vi "test_Read Cluster Register Value.vi"(8 "error in (no error)":errorcluster, 11 "TestCase in":refnum<class "FPGA Register IO Tests.lvclass">) -> (0 "error out":errorcluster, 3 "TestCase out":refnum<class "FPGA Register IO Tests.lvclass">)   [LabVIEW 2021, in "FPGA Register IO Tests.lvclass"]
uses:
  FPGA Register IO Tests.lvclass
  FPGA Register IO Tests.lvclass/FPGA Register IO Tests.ctl
  c83476ed-2beb-434a-be7f-ac9223862d10.vi
  APIs/FPGA Register IO/SubVIs/Parse Cluster Configuration.vi
  APIs/FPGA Register IO/Read Methods/Read Data Register/Instances/Read U8 Array.vi
  APIs/FPGA Register IO/SubVIs/Check Cluster Configuration Store.vi
  APIs/FPGA Register IO/Utilities/Find Register Offset.vi
  APIs/FPGA Register IO/SubVIs/Check Register Data Store.vi
  <userlib>/_OpenG.lib/lvdata/lvdata.llb/Variant to Header Info__ogtk.vi
  <userlib>/_OpenG.lib/lvdata/lvdata.llb/Split Cluster TD__ogtk.vi
  <userlib>/_OpenG.lib/lvdata/lvdata.llb/Cluster to Array of VData__ogtk.vi
  <vilib>/Utility/Data Type/Get Type Information.vi
  <userlib>/_OpenG.lib/lvdata/lvdata.llb/Get Strings from Enum__ogtk.vi
  APIs/FPGA Register IO/Error Handling/Error 6004.vi
  <vilib>/Utility/Data Type/Get Fixed-Point Information.vi
  APIs/FPGA Register IO/Error Handling/Error 6001.vi
  APIs/FPGA Register IO/Error Handling/Error 6000.vi
  APIs/FPGA Register IO/Error Handling/Error 6002.vi
  APIs/FPGA Register IO/Error Handling/Error 6003.vi
  <vilib>/FPGAPlugInAG/Dynamic/niLvFpga_Close_Dynamic.vi
  <vilib>/rvi/interface/nirviCloseFPGA/nirviCloseFPGA.xnode
  <vilib>/addons/_JKI Toolkits/VI Tester/TestCase.llb/TestCase.lvclass
  APIs/FPGA Register IO/FPGA Register IO.lvlib
  C:/Program Files/National Instruments/LabVIEW 2021/vi.lib/addons/_JKI Toolkits/VI Tester/TestCase.llb/TestCase.lvclass
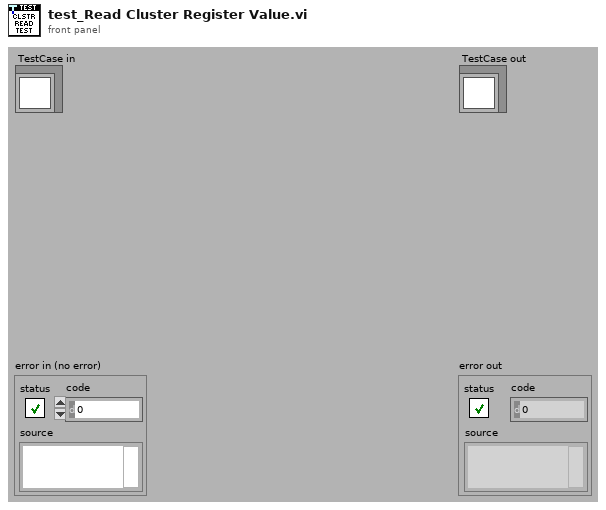
[diagram p1: front panel]
types:
  T1 = cluster{"I16":i16, "U64":u64, "SGL":sgl, "Bool":bool, "FXP 12/6":fxp<+/-,12,6>}
  T2 = cluster{"I16":i16, "U64":u64, "SGL":sgl, "Bool":bool, "FXP 12/6":fxp<+/-,12,6>}[]
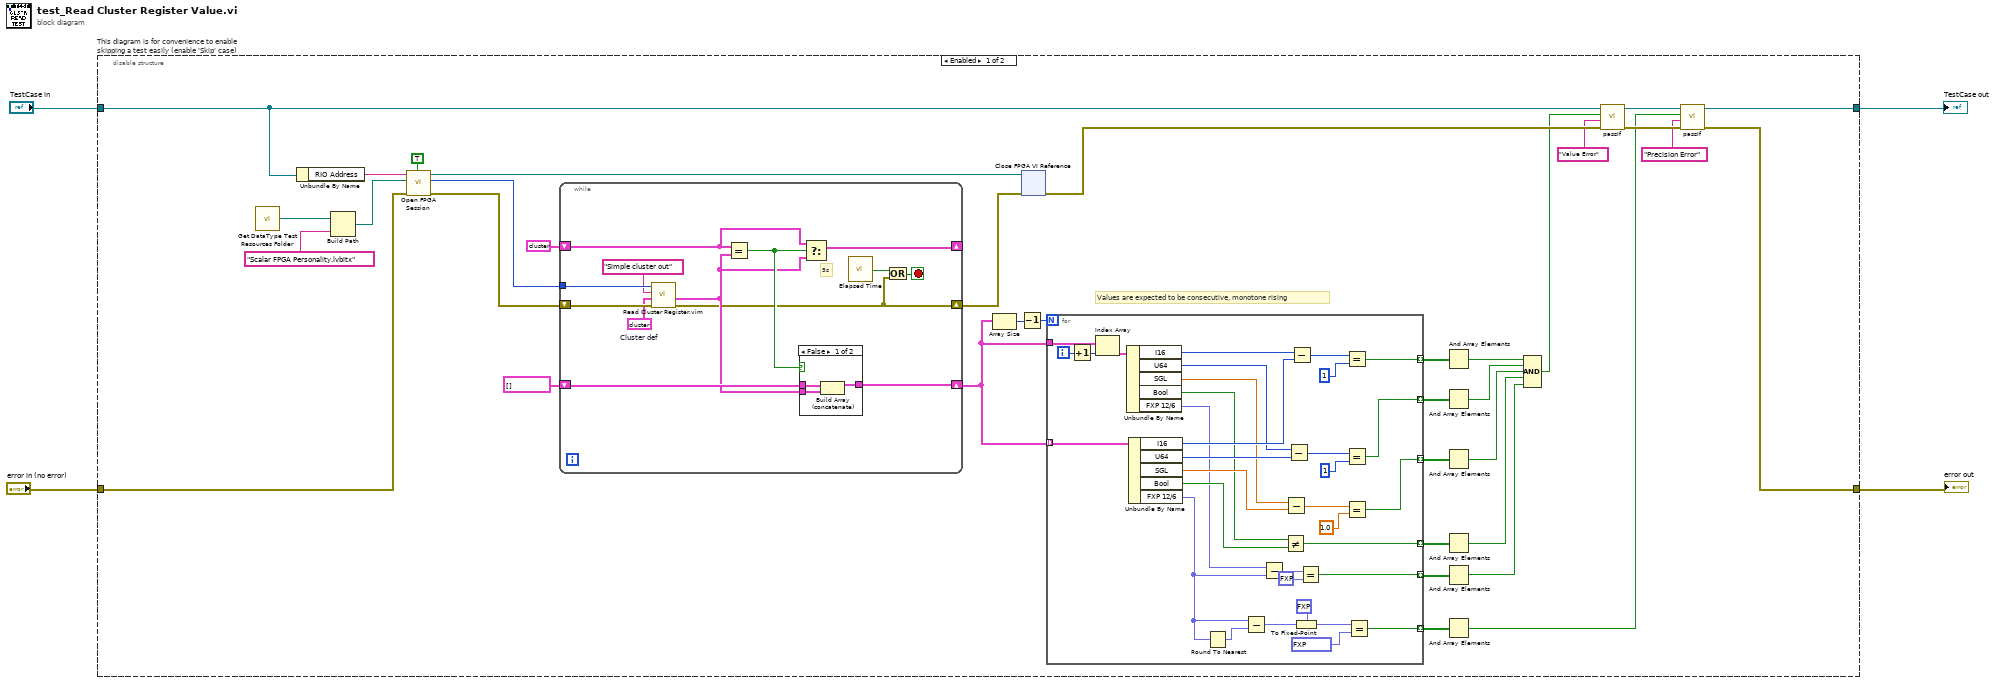
[diagram p0: block diagram]
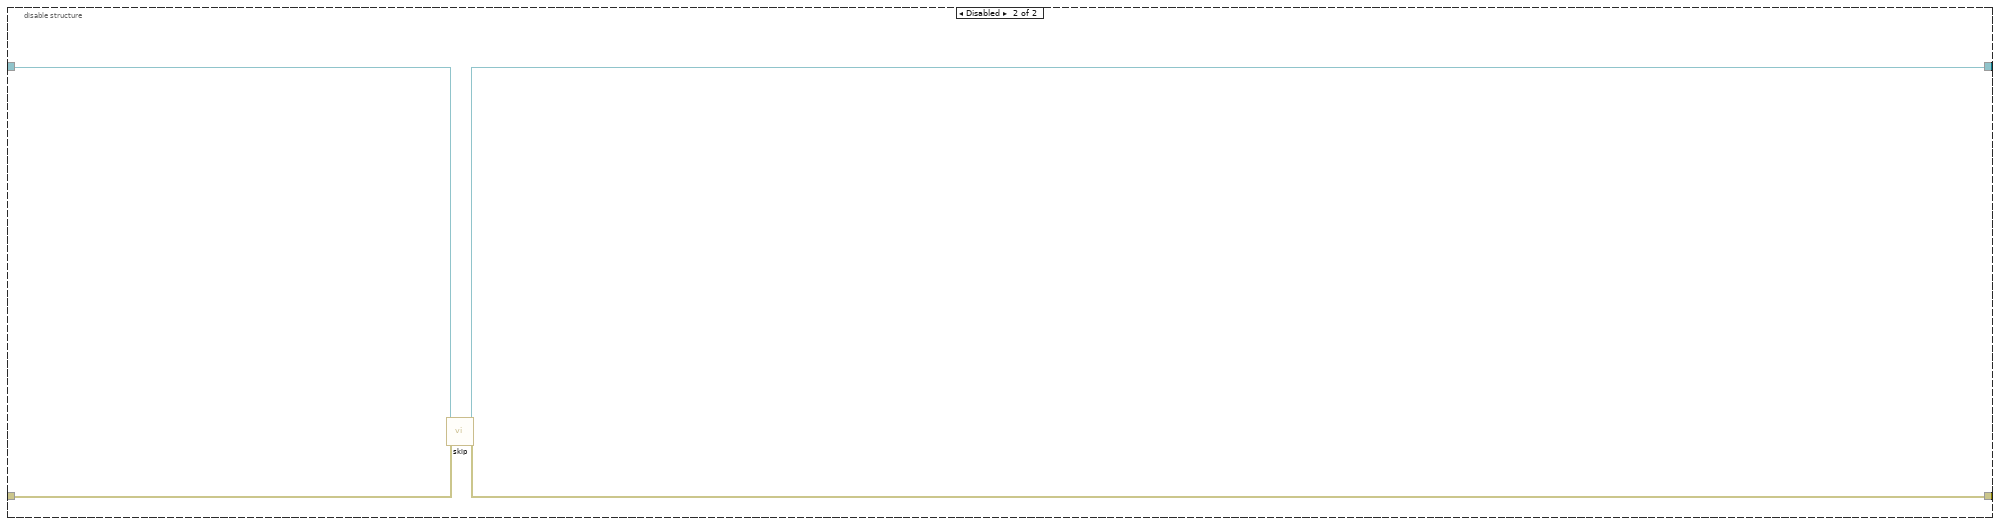
[diagram p3: hidden frame]
diagram:
  n1 = disable-structure "This diagram is for convenience to enable skipping a test easily (enable 'Skip' case)" shown="Enabled" {
    disable-tunnel: "TestCase in" -> [w31 w95]
    disable-tunnel: [w23 w93] -> w1
    disable-tunnel: [w24 w94] -> w3
    disable-tunnel: "error in (no error)" -> [w32 w92]
    frame Enabled {
      # "Values are expected to be consecutive, monotone rising"
      n2 = call "Get DataType Test Resources Folder.vi"() -> ("path"=w29:path)
      n3 = Unbundle By Name(w31) -> ("RIO Address"=w34:string)
      n4 = Build Path(base path=w29, name or relative path="Scalar FPGA Personality.lvbitx") -> (appended path=w33:path)
      n5 = call "Open FPGA Session.vi"("run when loaded (T)"=TRUE ("Run When Loaded (T)"), "error in"=w32, "bitfile path"=w33, "device address"=w34) -> ("error out"=w39:errorcluster, "session out"=w38:u32, "bitfile reference out"=w37:refnum<k20>)  [unwired: 5 in]
      n6 = while {
        tunnel: w38 -> [w81]
        shift-right: [w75] -> w36
        shift-left: w39 -> [w82]
        shift-right: [w86] -> _
        shift-left: T1 {"I16"=0, "U64"=0, "SGL"=0.0, "Bool"=FALSE, "FXP 12/6"=0.0} ("Cluster def") -> [w87]
        shift-right: [w76] -> w19
        shift-left: T2 [] -> [w85]
        stop <- w84 stop-if-true
        w80 = T1 {"I16"=0, "U64"=0, "SGL"=0.0, "Bool"=FALSE, "FXP 12/6"=0.0}  # Cluster def
        # "5s"
        n7 = call "Read Cluster Register.vim"("error in (no error)"=w82, "Cluster in (default value)"=w80, "Cluster Name"="Simple cluster out" ("registerName"), "session in"=w81) -> ("error out"=w75:errorcluster, "Cluster out"=w77:T1)  [unwired: 4 in, 2 out]
        n8 = Equal?(x=w87, y=w77) -> (x = y?=w78:bool)
        n9 = case shown="False" w78 {
          tunnel: [w90 w91] -> w76
          tunnel: w85 -> [w89 w91]
          tunnel: w77 -> [w88 _]
          frame False {
            n10 = Build Array (concatenate)(w89, w88) -> (w90:T2)
          }
          frame True {
          }
        }
        n11 = Select(t=w87, s=w78, f=w77) -> (s? t:f=w86:T1)
        n12 = call "Elapsed Time"() -> ("Time has Elapsed"=w83:bool)  [unwired: 12 in, 7 out]
        n13 = Or(x=w83, y=w75) -> (x .or. y?=w84:bool)
      }
      n14 = Array Size(array=w19) -> (size(s)=w17:i32)
      n15 = Decrement(x=w17) -> (x-1=w18:i32)
      n16 = xnode "Close FPGA VI Reference"("FPGA VI Reference In"=w37, "error in"=w36) -> ("error out"=w30:errorcluster)
      n17 = for {
        N: w18 -> [_]
        tunnel: w19 -> [w74] mode=indexing
        tunnel: w19 -> [w69]
        tunnel: [w65] -> w20 mode=indexing
        tunnel: [w60] -> w16 mode=indexing
        tunnel: [w55] -> w15 mode=indexing
        tunnel: [w52] -> w14 mode=indexing
        tunnel: [w48] -> w8 mode=indexing
        tunnel: [w41] -> w7 mode=indexing
        i -> [w70]
        n18 = Increment(x=w70) -> (x+1=w72:i32)
        n19 = Index Array(array=w69, index=w72) -> (element=w67:T1)
        n20 = Unbundle By Name(w67) -> ("I16"=w66:i16, "U64"=w61:u64, "SGL"=w56:sgl, "Bool"=w53:bool, "FXP 12/6"=w51:fxp<+/-,12,6>)
        n21 = Unbundle By Name(w74) -> ("I16"=w68:i16, "U64"=w62:u64, "SGL"=w57:sgl, "Bool"=w54:bool, "FXP 12/6"=w47:fxp<+/-,12,6>)
        n22 = Round To Nearest(number=w47) -> (nearest integer value=w46:fxp<+/-,7,7>)
        n23 = Subtract(x=w47, y=w46) -> (x-y=w45:fxp<+/-,13,7>)
        n24 = Subtract(x=w51, y=w47) -> (x-y=w50:fxp<+/-,13,7>)
        n25 = Not Equal?(x=w53, y=w54) -> (x != y?=w52:bool)
        n26 = Subtract(x=w56, y=w57) -> (x-y=w59:sgl)
        n27 = Subtract(x=w61, y=w62) -> (x-y=w63:u64)
        n28 = Subtract(x=w66, y=w68) -> (x-y=w73:i16)
        n29 = To Fixed-Point(fixed-point type=fxp<+/-,12,6> 0.0 ("FXP 12/6"), number=w45) -> (fixed-point=w43:fxp<+/-,12,6>)
        n30 = Equal?(x=w50, y=fxp<+/-,13,7> 1.0) -> (x = y?=w48:bool)
        n31 = Equal?(x=w73, y=i16 1) -> (x = y?=w65:bool)
        n32 = Equal?(x=w63, y=u64 1) -> (x = y?=w60:bool)
        n33 = Equal?(x=w59, y=sgl 1.0) -> (x = y?=w55:bool)
        n34 = Equal?(x=w43, y=fxp<+/-,12,6> 0.109375) -> (x = y?=w41:bool)
      }
      n35 = And Array Elements(Boolean array=w20) -> (logical AND=w13:bool)
      n36 = And Array Elements(Boolean array=w16) -> (logical AND=w12:bool)
      n37 = And Array Elements(Boolean array=w15) -> (logical AND=w11:bool)
      n38 = And Array Elements(Boolean array=w14) -> (logical AND=w10:bool)
      n39 = And Array Elements(Boolean array=w8) -> (logical AND=w6:bool)
      n40 = And Array Elements(Boolean array=w7) -> (logical AND=w5:bool)
      n41 = Compound Arithmetic op=AND(w13, w12, w11, w10, w6) -> (w9:bool)
      n42 = call-dynamic "passIf.vi"("error in (no error)"=w30, "message (\"\")"="Value Error" ("message (\"\")"), "pass"=w9, "TestCase in"=w31) -> ("error out"=w27:errorcluster, "TestCase out"=w26:refnum<class "FPGA Register IO Tests.lvclass">)  [unwired: 6 in]
      n43 = call-dynamic "passIf.vi"("error in (no error)"=w27, "message (\"\")"="Precision Error" ("message (\"\")"), "pass"=w5, "TestCase in"=w26) -> ("error out"=w24:errorcluster, "TestCase out"=w23:refnum<class "FPGA Register IO Tests.lvclass">)  [unwired: 6 in]
    }
    frame Disabled {
      # "skip test result while test is under development"
      n44 = call <vilib>:"skip.vi"("error in (no error)"=w92, "TestCase in"=w95) -> ("error out"=w94:errorcluster, "TestCase out"=w93:refnum<class "FPGA Register IO Tests.lvclass">)  [unwired: 8 in]
    }
  }
  "error out" <- w3
  "TestCase out" <- w1
